vi "Transmit.vi"(8 "error in (no error)":errorcluster, 11 "Framework in":refnum<class "Framework.lvclass">) -> (0 "error out":errorcluster, 3 "Framework out":refnum<class "Framework.lvclass">)   [LabVIEW 2017, in "DSF Core.lvlib" / "Framework.lvclass"]
uses:
  Framework.lvclass
  Framework.lvclass/Framework.ctl
  Performance/Performance.lvclass/Performance.ctl
  Plugin/Plugin.lvclass/Plugin.ctl
  Transfer Group/Transfer Group.lvclass/Transfer Group.ctl
  Timing/Timing.lvclass/Timing.ctl
  Buffers/Buffers.lvclass/Buffers.ctl
  <vilib>/NI/Memory Manager/Classes/Pointer/Pointer.lvclass/Pointer.ctl
  Interface/Interface.lvclass/Interface.ctl
  Transfer Group/Increment Iteration.vi
  Transfer Group/Copy Inline to Async.vi
  Transfer Group/Get Iteration.vi
  Thread/Dispatcher/Dispatch Transfer Group.vi
  Transfer Group/Get ID.vi
  Plugin/Get ID.vi
  Transfer Group/Wait For Previous.vi
  Transfer Group/Update Status.vi
  Transfer Group/Get Active.vi
  Timing/Increment Iteration.vi
  Buffers/Copy Inline to Async.vi
  Timing/Get Iteration.vi
  Interface/Dispatcher/Send Dispatcher Command.vi
  Transfer Group/Retrieve from FIFO.vi
  Status/Write Status.vi
  <vilib>/NI/Memory Manager/Classes/Pointer/Copy All.vi
  Interface/Dispatcher/Write.vi
  Interface/Dispatcher/Write Dispatcher Command.vi
  Transfer Group/Read Return FIFO.vi
  Transfer Group/Increment Late Count.vi
  <vilib>/NI/Memory Manager/Classes/Pointer/Get Address.vi
  Status/Status Size.vi
  <vilib>/NI/Memory Manager/Classes/Pointer/Check Null Pointer.vi
  <vilib>/NI/Memory Manager/Classes/Pointer/Check Size.vi
  <vilib>/NI/Memory Manager/Classes/Pointer/Get Size.vi
  <vilib>/NI/Memory Manager/Classes/Pointer/Copy.vi
  Interface/Send Command.vi
  <vilib>/NI/Memory Manager/Classes/Pointer/Errors.vi
  <vilib>/NI/Memory Manager/Classes/Pointer/Null Pointer.vi
  <vilib>/NI/Memory Manager/Classes/Pointer/Is Null.vi
  <vilib>/NI/Memory Manager/Classes/Pointer/Out of Bounds.vi
  <vilib>/NI/Memory Manager/Classes/Pointer/Copy (No Check).vi
  <vilib>/NI/Memory Manager/Classes/Pointer/Check Bounds (Pointer).vi
  Interface/Write RT FIFO.vi
  <vilib>/NI/Memory Manager/Classes/Pointer/Create Error.vi
  <vilib>/NI/Memory Manager/Classes/Pointer/Write Pointer Size to Error.vi
  <vilib>/NI/Memory Manager/Constants/Constants.vi
  <vilib>/NI/Memory Manager/Constants/Library Name.vi
  <vilib>/NI/Memory Manager/Classes/Pointer/Pointer Error Info.vi
  <vilib>/NI/Memory Manager/Constants/Pointer Class Name.vi
  Buffer/Buffer.lvclass
  C:/Program Files (x86)/National Instruments/LabVIEW 2017/vi.lib/NI/Memory Manager/Classes/Pointer/Pointer.lvclass
  Interface/Dispatcher/Dispatcher Interface.lvclass
  C:/Git/DSF/Core/Classes/Interface/Interface.lvclass
  Status/Status.lvclass
  <vilib>/NI/Memory Manager/VIs/Write String to Source.vi
  <vilib>/NI/Memory Manager/VIs/Write Numeric to Source.vi
  <vilib>/NI/Memory Manager/VIs/Write Numeric Scalar to Source (Base10 U64).vi
  <vilib>/NI/Memory Manager/VIs/Set Error Source.vi
  <vilib>/NI/Memory Manager/VIs/Set Error Code.vi
  <vilib>/NI/Memory Manager/VIs/Set Error Status.vi
  <vilib>/NI/Memory Manager/VIs/New Error Cluster.vi
  <vilib>/NI/Memory Manager/VIs/New Error Cluster (512B).vi
  Transfer Group/Errors.vi
  Transfer Group/Return Timeout Error.vi
  Transfer Group/Invalid Iteration Error.vi
  Interface/Errors.vi
  Interface/Dispatcher/Command Timeout.vi
  VIs/VI Name.vi
  Interface/Dispatcher/Class Name.vi
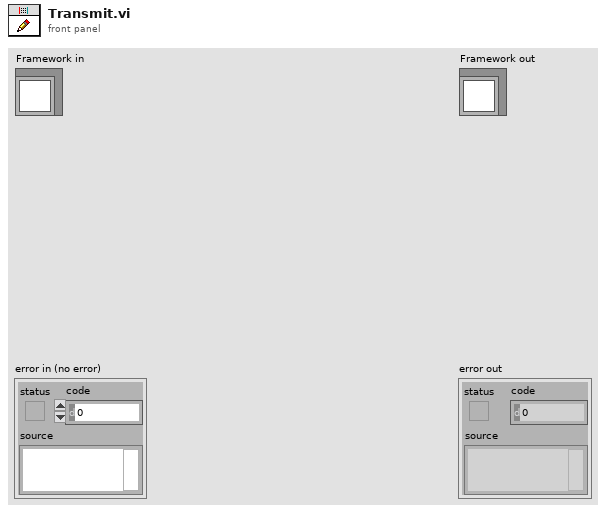
[diagram p1: front panel]
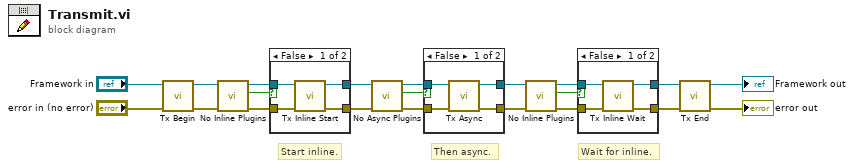
[diagram p0: block diagram]
diagram:
  # "Wait for inline."
  # "Start inline."
  # "Then async."
  n1 = call "Tx Begin.vi"("error in (no error)"="error in (no error)", "Framework in"="Framework in") -> ("error out"=w16:errorcluster, "Framework out"=w17:refnum<class "Framework.lvclass">)  [unwired: 8 in]
  n2 = call "No Inline Plugins.vi"("error in (no error)"=w16, "Framework in"=w17) -> ("error out"=w14:errorcluster, "no inline?"=w11:bool, "Framework out"=w15:refnum<class "Framework.lvclass">)  [unwired: 7 in]
  n3 = case shown="False" w11 {
    tunnel: w15 -> [w25 w27]
    tunnel: w14 -> [w24 w26]
    tunnel: [w23 w27] -> w13
    tunnel: [w22 w26] -> w12
    frame False {
      n4 = call "Tx Inline Start.vi"("error in (no error)"=w24, "Framework in"=w25) -> ("error out"=w22:errorcluster, "Framework out"=w23:refnum<class "Framework.lvclass">)  [unwired: 8 in]
    }
    frame True {
    }
  }
  n5 = call "No Async Plugins.vi"("error in (no error)"=w12, "Framework in"=w13) -> ("error out"=w10:errorcluster, "no async?"=w8:bool, "Framework out"=w9:refnum<class "Framework.lvclass">)  [unwired: 7 in]
  n6 = case shown="False" w8 {
    tunnel: w9 -> [w28 w33]
    tunnel: w10 -> [w29 w32]
    tunnel: [w30 w33] -> w4
    tunnel: [w31 w32] -> w3
    frame False {
      n7 = call "Tx Async.vi"("error in (no error)"=w29, "Framework in"=w28) -> ("error out"=w31:errorcluster, "Framework out"=w30:refnum<class "Framework.lvclass">)  [unwired: 8 in]
    }
    frame True {
    }
  }
  n8 = call "No Inline Plugins.vi"("error in (no error)"=w3, "Framework in"=w4) -> ("error out"=w7:errorcluster, "no inline?"=w5:bool, "Framework out"=w6:refnum<class "Framework.lvclass">)  [unwired: 7 in]
  n9 = case shown="False" w5 {
    tunnel: w6 -> [w34 w39]
    tunnel: w7 -> [w35 w38]
    tunnel: [w36 w39] -> w2
    tunnel: [w37 w38] -> w1
    frame False {
      n10 = call "Tx Inline Wait.vi"("error in (no error)"=w35, "Framework in"=w34) -> ("error out"=w37:errorcluster, "Framework out"=w36:refnum<class "Framework.lvclass">)  [unwired: 8 in]
    }
    frame True {
    }
  }
  n11 = call "Tx End.vi"("error in (no error)"=w1, "Framework in"=w2) -> ("error out"=→"error out":errorcluster, "Framework out"=→"Framework out":refnum<class "Framework.lvclass">)  [unwired: 8 in]
